vi "number1_global.vi"() -> ()   [LabVIEW 2014]
panel:
  in  "#s":dbl
  in  "Fs":dbl
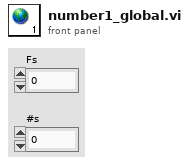
[diagram p1: front panel]
diagram:
